vi "SR FLip flop.vi"() -> ()   [LabVIEW 2021]
panel:
  in  "Clock":bool
  in  "R":bool
  in  "S":bool
  out "Q'":bool
  out "Q":bool
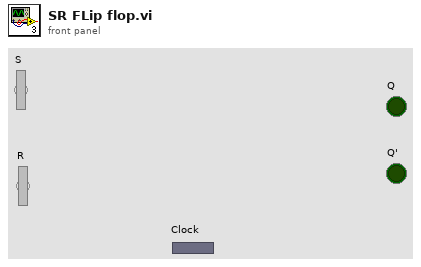
[diagram p1: front panel]
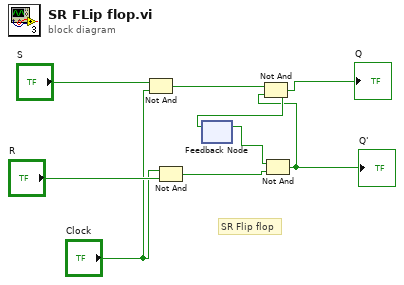
[diagram p0: block diagram]
diagram:
  # "SR Flip flop"
  n1 = Not And(1:"Clock", 2:"S") -> (0:w8:bool)
  n2 = Not And(1:"R", 2:"Clock") -> (0:w7:bool)
  n3 = feedback #1() -> (w6:bool)  [unwired: 1 in]
  n4 = Not And(1:w7, 2:w6) -> (0:w4:bool)
  "Q'" <- w4
  n5 = Not And(1:w4, 2:w8) -> (0:w5:bool)
  "Q" <- w5
  n6 = feedback-in #1(w5) -> ()
